vi "ProcessVision.vi"(0 "Image Src":T1, 1 "Min Radius":sgl=1.0 format="%.2f", 2 "Max Radius":sgl=10.0 format="%.2f", 3 "error in (no error)":errorcluster, 4 "RGB Cluster":cluster{"Red":T1, "Green":T1, "Blue":T1}) -> (5 "Image Out":T1, 6 "Circles Data":T2(array[cluster]), 7 "error out":errorcluster)   [LabVIEW 2013]
uses:
  <vilib>/vision/Image Controls.llb/IMAQ Image.ctl
  <vilib>/vision/NI_Vision_Development_Module.lvlib
panel:
  in  "Top of Range":i32
  in  "Bottom of Range":i32=480
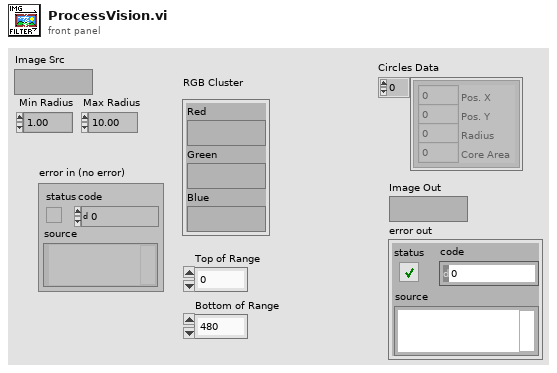
[diagram p1: front panel]
types:
  T1 = typedef "IMAQ Image.ctl" = refnum<image>
  T2 = cluster{"Pos. X":i32, "Pos. Y":i32, "Radius":i32, "Core Area":i32}[]
  T3 = typedef "Particle Parameters" = i32
  T4 = enum32{"AutoM", "Close", "Dilate", "Erode", "Gradient", "Gradient out", "Gradient in", "Hit miss", "Open", "PClose", "POpen", "Thick", "Thin"}
  T5 = cluster{"Measurement Parameter":T3, dbl, dbl, "Range":bool, "Measurement Type":bool}
  T6 = cluster{"Measurement Parameter":T3, dbl, dbl, "Range":bool, "Measurement Type":bool}[]
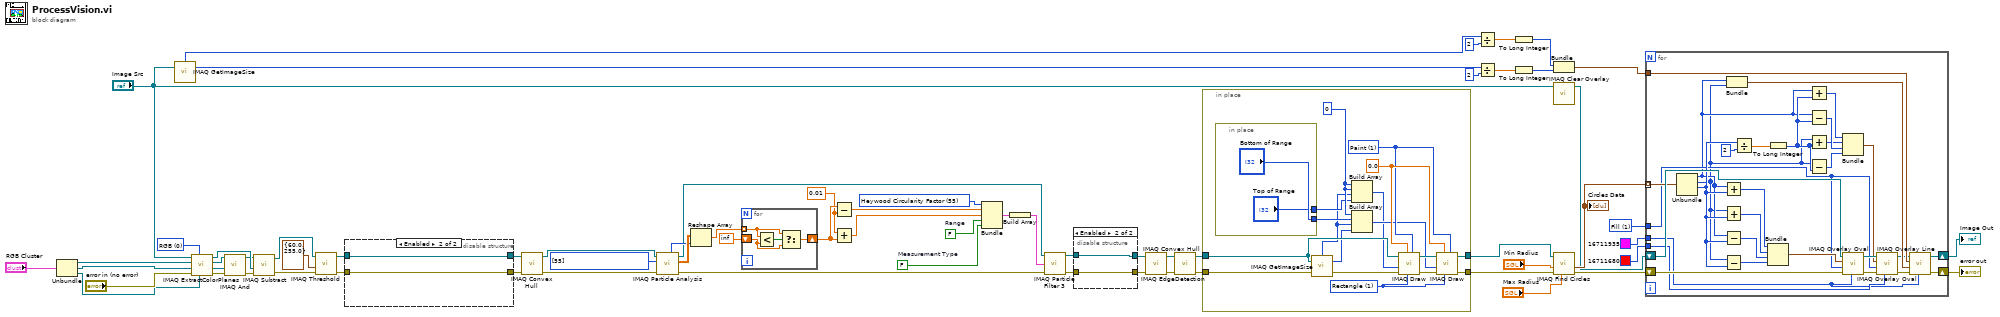
[diagram p0: block diagram]
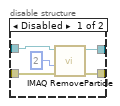
[diagram p2: hidden frame]
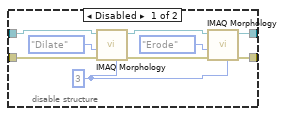
[diagram p3: hidden frame]
diagram:
  w7 = 0.01 ("x")
  w14 = FALSE  # Measurement Type
  w15 = FALSE  # Range
  w16 = T3 55 items=["Center of Mass X", "Center of Mass Y", "First Pixel X", "First Pixel Y", "Bounding Rect Left", "Bounding Rect Top", "Bounding Rect Right", "Bounding Rect Bottom", "Max Feret Diameter Start X", "Max Feret Diameter Start Y", "Max Feret Diameter End X", "Max Feret Diameter End Y", "Max Horiz. Segment Length Left", "Max Horiz. Segment Length Right", "Max Horiz. Segment Length Row", "-", "Bounding Rect Width", "Bounding Rect Height", "Bounding Rect Diagonal", "Perimeter", "Convex Hull Perimeter", "Holes' Perimeter", "Max Feret Diameter", "Equivalent Ellipse Major Axis", "Equivalent Ellipse Minor Axis", "Equivalent Ellipse Minor Axis (Feret)", "Equivalent Rect Long Side", "Equivalent Rect Short Side", "Equivalent Rect Diagonal", "Equivalent Rect Short Side (Feret)", "Average Horiz. Segment Length", "Average Vert. Segment Length", "Hydraulic Radius", "Waddel Disk Diameter", "-", "Area", "Holes' Area", "Particle & Holes' Area", "Convex Hull Area", "Image Area", "-", "Number of Holes", "Number of Horiz. Segments", "Number of Vert. Segments", "-", "Orientation", "Max Feret Diameter Orientation", "-", "% Area/Image Area", "% Area/(Particle & Holes' Area)", "Ratio of Equivalent Ellipse Axes", "Ratio of Equivalent Rect Sides", "-", "Elongation Factor", "Compactness Factor", "Heywood Circularity Factor", "Type Factor", "-", "Sum X", "Sum Y", "Sum XX", "Sum XY", "Sum YY", "Sum XXX", "Sum XXY", "Sum XYY", "Sum YYY", "-", "Moment of Inertia XX", "Moment of Inertia XY", "Moment of Inertia YY", "Moment of Inertia XXX", "Moment of Inertia XXY", "Moment of Inertia XYY", "Moment of Inertia YYY", "Norm. Moment of Inertia XX", "Norm. Moment of Inertia XY", "Norm. Moment of Inertia YY", "Norm. Moment of Inertia XXX", "Norm. Moment of Inertia XXY", "Norm. Moment of Inertia XYY", "Norm. Moment of Inertia YYY", "Hu Moment 1", "Hu Moment 2", "Hu Moment 3", "Hu Moment 4", "Hu Moment 5", "Hu Moment 6", "Hu Moment 7"] ("Measurement Parameter")
  w18 = T3[] [55] items=["Center of Mass X", "Center of Mass Y", "First Pixel X", "First Pixel Y", "Bounding Rect Left", "Bounding Rect Top", "Bounding Rect Right", "Bounding Rect Bottom", "Max Feret Diameter Start X", "Max Feret Diameter Start Y", "Max Feret Diameter End X", "Max Feret Diameter End Y", "Max Horiz. Segment Length Left", "Max Horiz. Segment Length Right", "Max Horiz. Segment Length Row", "-", "Bounding Rect Width", "Bounding Rect Height", "Bounding Rect Diagonal", "Perimeter", "Convex Hull Perimeter", "Holes' Perimeter", "Max Feret Diameter", "Equivalent Ellipse Major Axis", "Equivalent Ellipse Minor Axis", "Equivalent Ellipse Minor Axis (Feret)", "Equivalent Rect Long Side", "Equivalent Rect Short Side", "Equivalent Rect Diagonal", "Equivalent Rect Short Side (Feret)", "Average Horiz. Segment Length", "Average Vert. Segment Length", "Hydraulic Radius", "Waddel Disk Diameter", "-", "Area", "Holes' Area", "Particle & Holes' Area", "Convex Hull Area", "Image Area", "-", "Number of Holes", "Number of Horiz. Segments", "Number of Vert. Segments", "-", "Orientation", "Max Feret Diameter Orientation", "-", "% Area/Image Area", "% Area/(Particle & Holes' Area)", "Ratio of Equivalent Ellipse Axes", "Ratio of Equivalent Rect Sides", "-", "Elongation Factor", "Compactness Factor", "Heywood Circularity Factor", "Type Factor", "-", "Sum X", "Sum Y", "Sum XX", "Sum XY", "Sum YY", "Sum XXX", "Sum XXY", "Sum XYY", "Sum YYY", "-", "Moment of Inertia XX", "Moment of Inertia XY", "Moment of Inertia YY", "Moment of Inertia XXX", "Moment of Inertia XXY", "Moment of Inertia XYY", "Moment of Inertia YYY", "Norm. Moment of Inertia XX", "Norm. Moment of Inertia XY", "Norm. Moment of Inertia YY", "Norm. Moment of Inertia XXX", "Norm. Moment of Inertia XXY", "Norm. Moment of Inertia XYY", "Norm. Moment of Inertia YYY", "Hu Moment 1", "Hu Moment 2", "Hu Moment 3", "Hu Moment 4", "Hu Moment 5", "Hu Moment 6", "Hu Moment 7"] ("Pixel Measurements")
  w60 = u32 1 items=["Frame", "Fill"] ("Drawing Mode (Frame)")
  w66 = u16 0 items=["RGB", "HSL", "HSV", "HSI"] ("Color Mode")
  n1 = Unbundle("RGB Cluster") -> ("Red"=w41:T1, "Green"=w40:T1, "Blue"=w39:T1)
  n2 = call "IMAQ GetImageSize"("Image"="Image Src") -> ("Y Resolution"=w32:i32, "X Resolution"=w35:i32)  [unwired: 3 in, 1 out]
  n3 = call "IMAQ ExtractColorPlanes"("Blue or Luma or Val or Inten Plane"=w39, "Color Mode"=w66, "error in (no error)"="error in (no error)", "Green or Sat Plane"=w40, "Red or Hue Plane"=w41, "Image Src"="Image Src") -> ("error out"=w38:errorcluster, "Blue or Luma or Val or Inten Plane out"=w55:T1, "Green or Sat Plane out"=w56:T1, "Red or Hue Plane out"=w54:T1)  [unwired: 2 in]
  n4 = call "IMAQ And"("error in (no error)"=w38, "Image Src B"=w55, "Image Src A"=w56) -> ("error out"=w47:errorcluster, "Image Dst Out"=w48:T1)  [unwired: 7 in]
  n5 = call "IMAQ Subtract"("Image Src A"=w48, "Image Src B"=w54, "error in (no error)"=w47) -> ("Image Dst Out"=w44:T1, "error out"=w43:errorcluster)  [unwired: 4 in]
  n6 = call "IMAQ Threshold"("error in (no error)"=w43, "Range"=cluster{"Lower value":sgl, "Upper value":sgl} {"Lower value"=60.0, "Upper value"=255.0}, "Image Src"=w44) -> ("error out"=w46:errorcluster, "Image Dst Out"=w45:T1)  [unwired: 7 in]
  n7 = disable-structure shown="Enabled" {
    disable-tunnel: [w71 w77] -> w52
    disable-tunnel: [w70 w78] -> w51
    disable-tunnel: w46 -> [w69 w77]
    disable-tunnel: w45 -> [w68 w78]
    frame Disabled {
      w73 = 3 ("Number of iterations (1)")
      n8 = call "IMAQ Morphology"("Number of iterations (1)"=w73, "error in (no error)"=w69, "Operation"=T4."Dilate", "Image Src"=w68) -> ("error out"=w74:errorcluster, "Image Dst Out"=w75:T1)  [unwired: 6 in]
      n9 = call "IMAQ Morphology"("Number of iterations (1)"=w73, "error in (no error)"=w74, "Operation"=T4."Erode", "Image Src"=w75) -> ("error out"=w71:errorcluster, "Image Dst Out"=w70:T1)  [unwired: 6 in]
    }
    frame Enabled {
    }
  }
  n10 = call "IMAQ Convex Hull"("error in (no error)"=w52, "Image Src"=w51) -> ("error out"=w2:errorcluster, "Image Dst Out"=w17:T1)  [unwired: 8 in]
  n11 = call "IMAQ Particle Analysis"("error in (no error)"=w2, "Pixel Measurements"=w18, "Image"=w17) -> ("error out"=w1:errorcluster, "Particle Measurements (Pixels)"=w10:dbl[][], "Image Out (duplicate)"=w3:T1, "Number of Particles"=w4:i32)  [unwired: 3 in, 2 out]
  n12 = Reshape Array(w10, w4) -> (w9:dbl[])
  n13 = for {
    tunnel: w9 -> [w81] mode=indexing
    shift-right: [w79] -> w8
    shift-left: inf -> [w80]
    n14 = Less?(x=w81, y=w80) -> (x < y?=w82:bool)
    n15 = Select(t=w81, s=w82, f=w80) -> (s? t:f=w79:dbl)
  }
  n16 = Subtract(x=w8, y=w7) -> (x-y=w5:dbl)
  n17 = Add(x=w7, y=w8) -> (x+y=w6:dbl)
  n18 = Bundle("Measurement Parameter"=w16, w5, w6, "Range"=w15, "Measurement Type"=w14) -> (w13:T5)  [unwired: 1 in]
  n19 = Build Array(w13) -> (w12:T6)
  n20 = call "IMAQ Particle Filter 3"("Image Src"=w3, "Selection Values"=w12, "error in (no error)"=w1) -> ("Image Dst Out"=w22:T1, "error out"=w21:errorcluster)  [unwired: 10 in, 1 out]
  n21 = disable-structure shown="Enabled" {
    disable-tunnel: w22 -> [w86 w89]
    disable-tunnel: w21 -> [w85 w88]
    disable-tunnel: [w84 w88] -> w20
    disable-tunnel: [w83 w89] -> w19
    frame Disabled {
      n22 = call "IMAQ RemoveParticle"("error in (no error)"=w85, "Number of Erosion"=2, "Image Src"=w86) -> ("error out"=w84:errorcluster, "Image Dst Out"=w83:T1)  [unwired: 7 in]
    }
    frame Enabled {
    }
  }
  n23 = call "IMAQ EdgeDetection"("error in (no error)"=w20, "Image Src"=w19) -> ("error out"=w49:errorcluster, "Image Dst Out"=w50:T1)  [unwired: 8 in]
  n24 = call "IMAQ Convex Hull"("error in (no error)"=w49, "Image Src"=w50) -> ("error out"=w24:errorcluster, "Image Dst Out"=w23:T1)  [unwired: 8 in]
  n25 = in-place {
    in-place-border: [w105] -> w26
    in-place-border: [w100] -> w25
    in-place-border: w24 -> [w99]
    in-place-border: w23 -> [w97]
    w95 = 0
    w102 = u16 1 items=["Line", "Rectangle", "Oval"] ("Shape to draw")
    w104 = sgl 0.0 ("Pixel Color")
    w103 = u16 1 items=["Frame", "Paint", "Invert Frame", "Invert Paint"] ("Draw Mode")
    n26 = in-place {
      in-place-border: ["Bottom of Range"] -> w96
      in-place-border: ["Top of Range"] -> w94
    }
    n27 = call "IMAQ GetImageSize"("Image"=w97, "error in (no error)"=w99) -> ("Y Resolution"=w92:i32, "X Resolution"=w93:i32, "error out"=w98:errorcluster)  [unwired: 2 in]
    n28 = Build Array(w95, w95, w93, w94) -> (w90:i32[])
    n29 = Build Array(w95, w96, w93, w92) -> (w91:i32[])
    n30 = call "IMAQ Draw"("Draw Mode"=w103, "Shape to draw"=w102, "Pixel Color"=w104, "error in (no error)"=w98, "Coordinates"=w90, "Image Src"=w97) -> ("error out"=w101:errorcluster, "Image Dst Out"=w106:T1)  [unwired: 4 in]
    n31 = call "IMAQ Draw"("Draw Mode"=w103, "Shape to draw"=w102, "Pixel Color"=w104, "error in (no error)"=w101, "Coordinates"=w91, "Image Src"=w106) -> ("error out"=w100:errorcluster, "Image Dst Out"=w105:T1)  [unwired: 4 in]
  }
  n32 = Divide(x=w35, y=2) -> (x/y=w30:dbl)
  n33 = Divide(x=w32, y=2) -> (x/y=w31:dbl)
  n34 = To Long Integer(number=w30) -> (32bit integer=w29:i32)
  n35 = To Long Integer(number=w31) -> (32bit integer=w28:i32)
  n36 = Bundle(w29, w28) -> (w27:cluster{i32, i32})  [unwired: 1 in]
  n37 = call "IMAQ Clear Overlay"("Image"="Image Src") -> ("Image Out"=w62:T1)  [unwired: 9 in, 1 out]
  n38 = call "IMAQ Find Circles"("Max Radius"="Max Radius", "error in (no error)"=w25, "Min Radius"="Min Radius", "Image Src"=w26) -> ("error out"=w61:errorcluster, "Circles Data"=w63:T2)  [unwired: 4 in, 2 out]
  "Circles Data" <- w63
  n39 = for {
    tunnel: w63 -> [w136] mode=indexing
    shift-right: [w111] -> w58
    shift-left: w62 -> [w138]
    tunnel: w60 -> [w119]
    tunnel: u32 16711935 ("Color") -> [w109]
    shift-right: [w110] -> w57
    shift-left: w61 -> [w137]
    tunnel: u32 16711680 ("Color") -> [w118]
    tunnel: w27 -> [w117]
    n40 = Unbundle(w136) -> ("Pos. X"=w116:i32, "Pos. Y"=w115:i32, "Radius"=w126:i32)  [unwired: 1 out]
    n41 = Add(x=w116, y=w126) -> (x+y=w135:i32)
    n42 = Add(x=w115, y=w126) -> (x+y=w134:i32)
    n43 = Subtract(x=w116, y=w126) -> (x-y=w133:i32)
    n44 = Subtract(x=w115, y=w126) -> (x-y=w132:i32)
    n45 = Bundle("Pos. X"=w116, "Pos. Y"=w115) -> (w114:cluster{"Pos. X":i32, "Pos. Y":i32})  [unwired: 1 in]
    n46 = Divide(x=w126, y=2) -> (x/y=w124:dbl)
    n47 = To Long Integer(number=w124) -> (32bit integer=w123:i32)
    n48 = Bundle(w135, w134, w133, w132) -> (w131:cluster{i32, i32, i32, i32})  [unwired: 1 in]
    n49 = Add(x=w116, y=w123) -> (x+y=w127:i32)
    n50 = Subtract(x=w116, y=w123) -> (x-y=w129:i32)
    n51 = Add(x=w115, y=w123) -> (x+y=w128:i32)
    n52 = Subtract(x=w115, y=w123) -> (x-y=w130:i32)
    n53 = Bundle(w127, w128, w129, w130) -> (w120:cluster{i32, i32, i32, i32})  [unwired: 1 in]
    n54 = call "IMAQ Overlay Oval"("Color"=w109, "error in (no error)"=w137, "Drawing Mode (Frame)"=w119, "Bounding Rectangle"=w131, "Image"=w138) -> ("error out"=w121:errorcluster, "Image Out"=w122:T1)  [unwired: 5 in]
    n55 = call "IMAQ Overlay Oval"("Color"=w118, "error in (no error)"=w121, "Drawing Mode (Frame)"=w119, "Bounding Rectangle"=w120, "Image"=w122) -> ("error out"=w113:errorcluster, "Image Out"=w112:T1)  [unwired: 5 in]
    n56 = call "IMAQ Overlay Line"("Color"=w109, "error in (no error)"=w113, "End Point"=w114, "Start Point"=w117, "Image"=w112) -> ("error out"=w110:errorcluster, "Image Out"=w111:T1)  [unwired: 5 in]
  }
  "Image Out" <- w58
  "error out" <- w57
